vi "Get VeriStand Common Directory.vi"() -> (3 "common directory":path)   [LabVIEW 2019, in "DSF System Explorer.lvlib"]
uses:
  DSF System Explorer.lvlib
  NationalInstruments.VeriStand.Internal
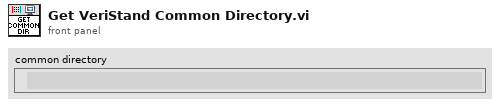
[diagram p1: front panel]
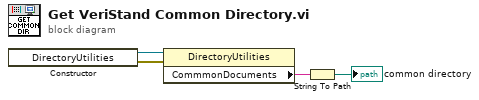
[diagram p0: block diagram]
diagram:
  n1 = constructor class="DirectoryUtilities"() -> (reference out=w4:refnum<k24>, error out=w3:errorcluster)  [unwired: 3 in, 1 out]
  n2 = property class="DirectoryUtilities"(reference=w4, error in=w3) -> ("CommmonDocuments"=w2:string)  [unwired: 2 out]
  n3 = String To Path(string=w2) -> (path=→"common directory":path)
